vi "Find Resources.vi"() -> ()   [LabVIEW 2014]
uses:
  <vilib>/MakerHub/LINX/LMH-LINX.lvlib
  <vilib>/MakerHub/LINX/Public/Utilities/Open Local.vi
  <vilib>/MakerHub/LINX/Public/Peripherals/UART/UART Read String.vi
panel:
  out "Device Name":string
  out "Data":string
  in  "stop":bool
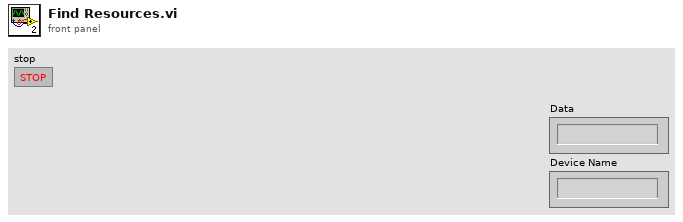
[diagram p1: front panel]
types:
  T1 = typedef "LMH-LINX.lvlib/LINX Ref.ctl" = cluster{"IO":T2, "Interface":T3, "LINX Device Config":T4}
  T2 = typedef "LMH-LINX.lvlib/Platform.ctl" = enum16{"Remote", "Local"}
  T3 = typedef "LMH-LINX.lvlib/Interface.ctl" = enum16{"Serial", "TCP"}
  T4 = typedef "LMH-LINX.lvlib/Device.lvlib/LINX Device Config.ctl" = cluster{"Interface":T3, "COM Port":refnum<visa-resource-name>, "TCP Configuration":T5, "Device Family":u8, "Device ID":u8, "Device Name":string, "TCP Ref":refnum<k5>, "Channels":T6}
  T5 = typedef "LMH-LINX.lvlib/Device.lvlib/TCP Config.ctl" = cluster{"IP Address":string, "Port":u16}
  T6 = typedef "LMH-LINX.lvlib/Channels.ctl" = cluster{"DI":u8[], "DO":u8[], "AI":u8[], "AO":u8[], "PWM":u8[], "QE":u8[], "UART":u8[], "I2C 2":u8[], "SPI":u8[], "CAN":u8[], "Servo":u8[], "AI Ref (V)":dbl, "AI Resolution (Bits)":u8, "AO Ref (V)":dbl, "AO Resolution (Bits)":u8}
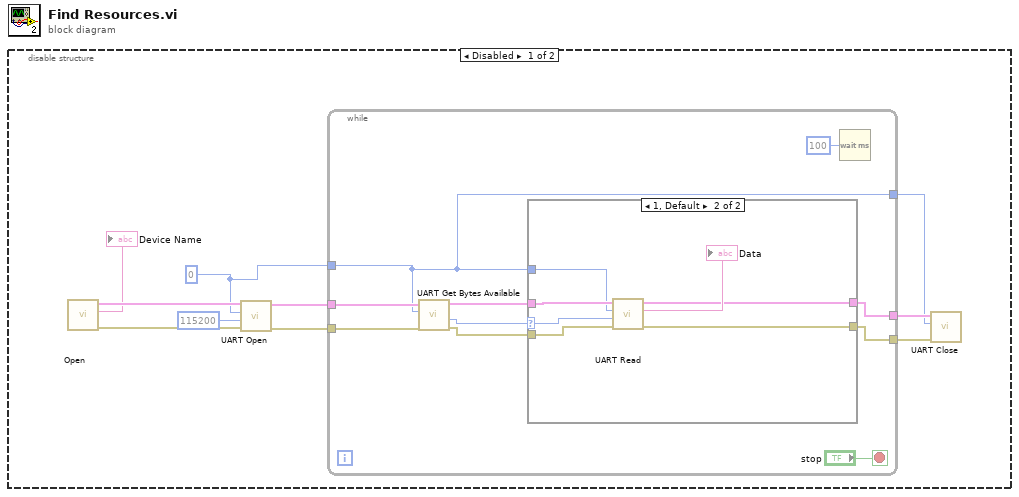
[diagram p0: block diagram]
diagram:
  n1 = disable-structure shown="Disabled" {
    frame Disabled {
      w5 = u8 0 ("UART Channel (0)")
      n2 = call-poly <vilib>:"Open.vi"() -> ("Error Out"=w9:errorcluster, "Device Name"=→"Device Name":string, "LINX Resource"=w10:T1)  [unwired: 9 in]
      n3 = call <vilib>:"UART Open.vi"("Error In"=w9, "Baud Rate (9600)"=u32 115200, "UART Channel (0)"=w5, "LINX Resource"=w10) -> ("Error Out"=w7:errorcluster, "LINX Resource"=w6:T1)  [unwired: 5 in, 1 out]
      n4 = while {
        tunnel: w7 -> [w20]
        tunnel: w6 -> [w19]
        tunnel: w5 -> [w12]
        tunnel: [w14] -> w4
        tunnel: [w13] -> w3
        tunnel: [w12] -> w2
        stop <- "stop" stop-if-true
        n5 = call <vilib>:"UART Get Bytes Available.vi"("Error In"=w20, "UART Channel (0)"=w12, "LINX Resource"=w19) -> ("Error Out"=w15:errorcluster, "Bytes Available"=w17:u8, "LINX Resource"=w16:T1)  [unwired: 6 in]
        n6 = case shown="1, Default" w17 {
          selector: w17 -> [_ w27]
          tunnel: w16 -> [w22 w28]
          tunnel: w15 -> [w21 w29]
          tunnel: w12 -> [_ w26]
          tunnel: [w21 w24] -> w13
          tunnel: [w22 w23] -> w14
          frame 0 {
          }
          frame 1, Default {
            n7 = call-poly <vilib>:"UART Read.vi"("Error In"=w29, "Num Bytes"=w27, "UART Channel (0)"=w26, "LINX Resource"=w28) -> ("Error Out"=w24:errorcluster, "Data"=→"Data":string, "LINX Resource"=w23:T1)  [unwired: 5 in]
          }
        }
        n8 = Wait (ms)(milliseconds to wait=u32 100) -> ()  [unwired: 1 out]
      }
      n9 = call <vilib>:"UART Close.vi"("Error In"=w3, "UART Channel (0)"=w2, "LINX Resource"=w4) -> ()  [unwired: 7 in, 2 out]
    }
    frame Enabled {
    }
  }
